vi "Dialog.vi"(8 "error in (no error)":errorcluster, 10 "Scripts Dir":path, 11 "Definitions in":T1) -> (0 "error out":errorcluster, 2 "commit?":bool, 3 "Definitions out":T1)   [LabVIEW 2019, in "Script.lvlib"]
doc: "Help dialog to configure script shortctus.\n\nCreated by: Ryan Pacini"
uses:
  Script.lvlib
  Definitions.ctl
panel:
  in  "open_qd_vi":bool
  in  "Cancel":bool
  in  "OK":bool
  in  "tab":enum32{"Help", "Script Shortcuts"}(tab)
  in  "info":string="Instructions:\n  Enter one or more script shortcuts (separated by a space) into\n  the Quick Drop textbox to execute a series of actions on the\n  selected front panel or block diagram objects.\n\nUsage: Ctrl-Space + \"<shortcut>\" + Ctrl-S"
  in  "Script Help":u16(ring) items=["Select VI...", "Builtins.vi", "TestScript.vi"]
  out "Description":string
  out "Scripts:":string
  in  "Show VI Info":bool
  in  "Shortcut":string
  in  "Action":u16(ring) items=["None", "Align Bottom Edges", "Align Horizontal Centers", "Align Left Edges", "Align Right Edges", "Align Top Edges", "Align Vertical Centers", "Arrange", "Change to CDB", "Change to CSG", "Change to CXT", "Change to DBL", "Change to EXT", "Change to I16", "Change to I32", "Change to I64", "Change to I8", "Change to SGL", "Change to U16", "Change to U32", "Change to U64", "Change to U8", "Cluster Size Fit", "Cluster Size Horizontally", "Cluster Size None", "Cluster Size Vertically", "Connect Pane", "Distribute Bottom Edges", "Distribute Horizontal Centers", "Distribute Horizontal Compress", "Distribute Horizontal Gap", "Distribute Left Edges", "Distribute Right Edges", "Distribute Top Edges", "Distribute Vertical Centers", "Distribute Vertical Compress", "Distribute Vertical Gap", "Edit Library Icon", "Error Structure", "Hide Caption", "Hide Inc/Dec Buttons", "Hide Index Display", "Hide Label", "Hide Radix", "Hide Scrollbars", "Merge Icon Layers", "My Custom Shortcut", "My Custom Shortcut with Args", "Open in File Explore", "Radix Binary or Backslash", "Radix Decimal or Normal", "Radix Hex", "Rename Caption", "Rename Label", "Reset Panel Origins", "Resizes Window", "Select Controls", "Select Controls and Indicators", "Select Indicators", "Select None", "Show Caption", "Show Inc/Dec Buttons", "Show Index Display", "Show Label", "Show Scrollbars", "Snap to Panel Grid", "VI Voodoo"]
  in  "add":bool
  in  "Script Shortcuts":i32[](listbox)
  in  "remove_shortcuts":bool
  in  "remove_all":bool
  in  "restore_defaults":bool
  in  "remove_action":bool
  in  "Actions":i32(listbox)
  in  "move_up":bool
  in  "move_down":bool
  # "Add Shortcut"
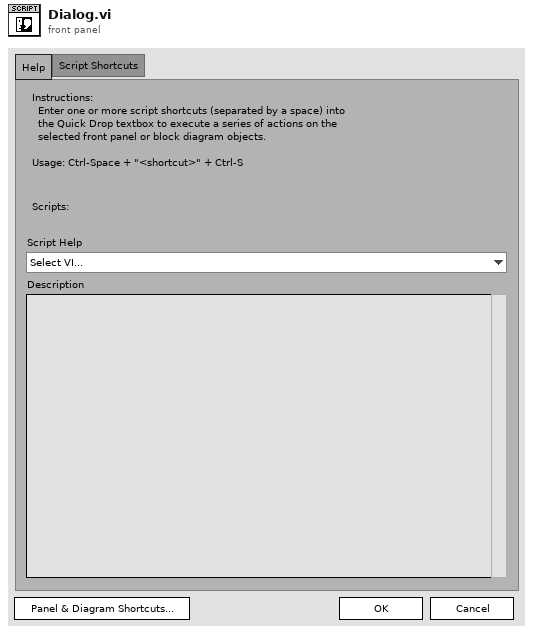
[diagram p1: front panel]
types:
  T1 = typedef "Script.lvlib/Definitions.ctl" = cluster{"plugins":cluster{"vi":path, "desc":string}[], "defaults":cluster{"uid":string, "name":string}[], "shortcuts":cluster{"shortcut":string, "uids":string[]}[], "defaults?":bool}
  T2 = cluster{"defs":T1, "ScriptsDir":path, "_sc":string, "_uid":string, "_show_uids":bool, "_action_idx":i32}
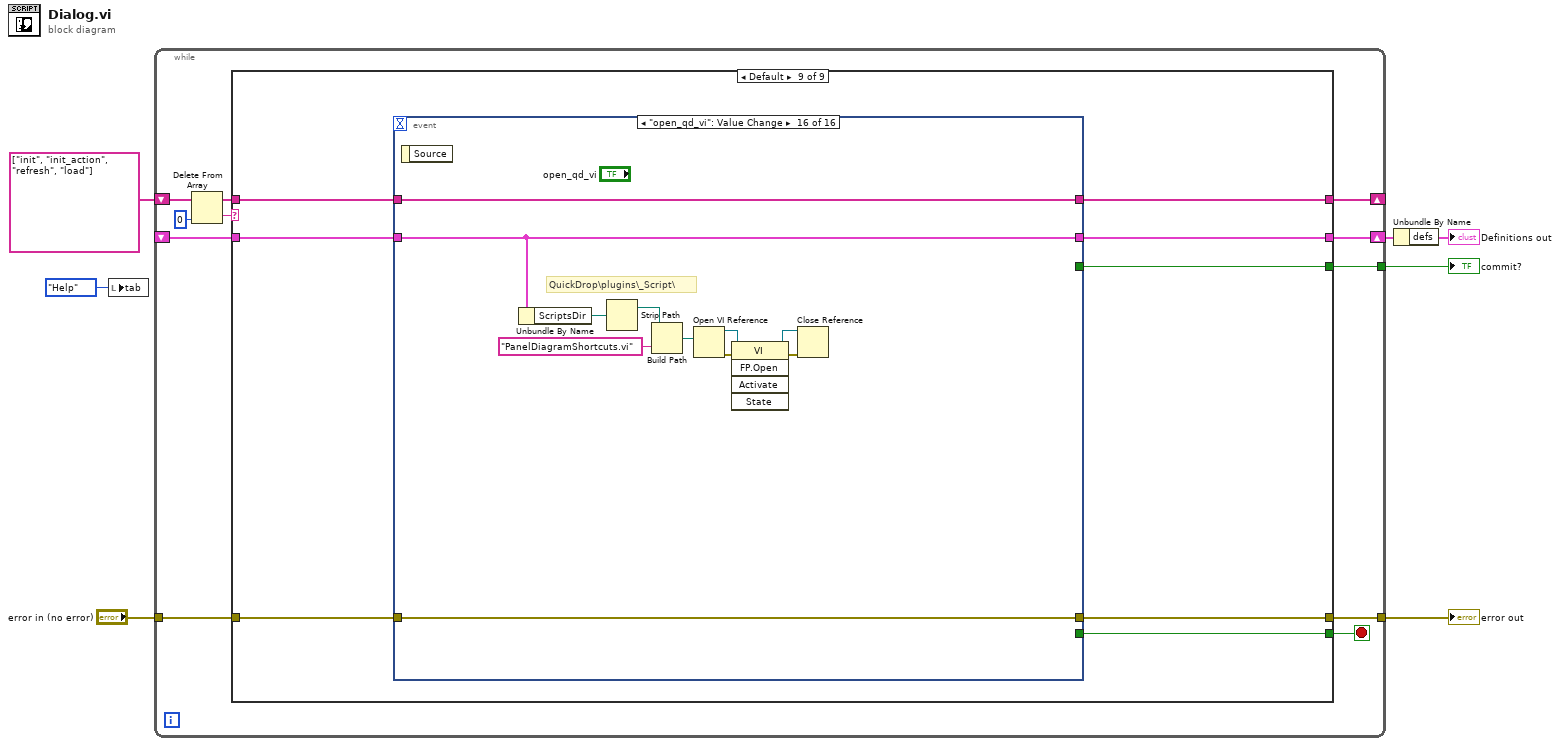
[diagram p0: block diagram]
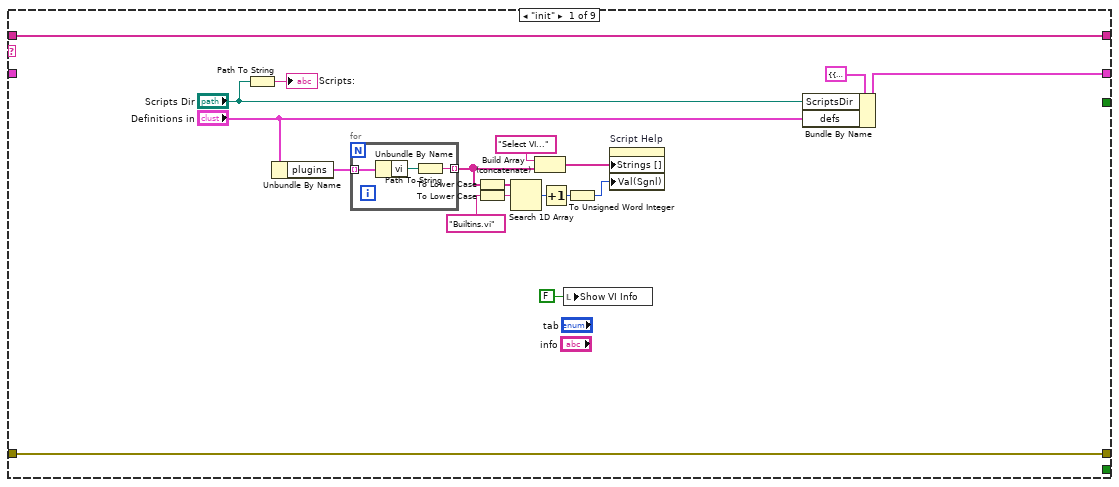
[diagram p2: hidden frame]
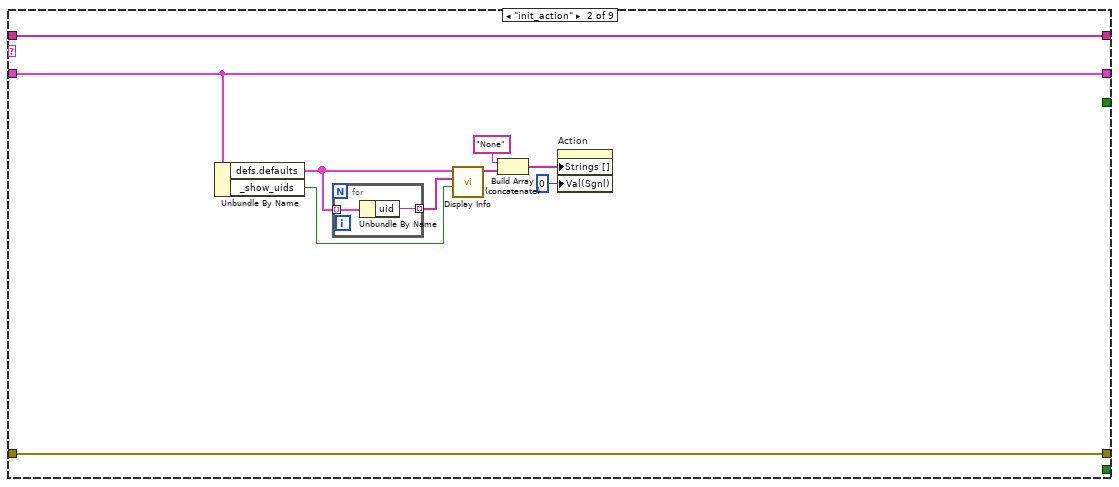
[diagram p3: hidden frame]
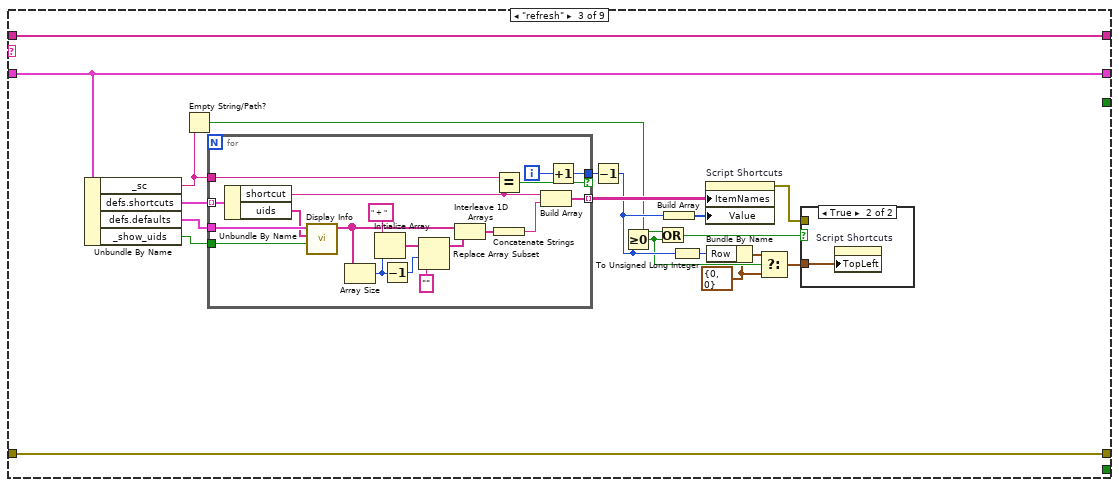
[diagram p4: hidden frame]
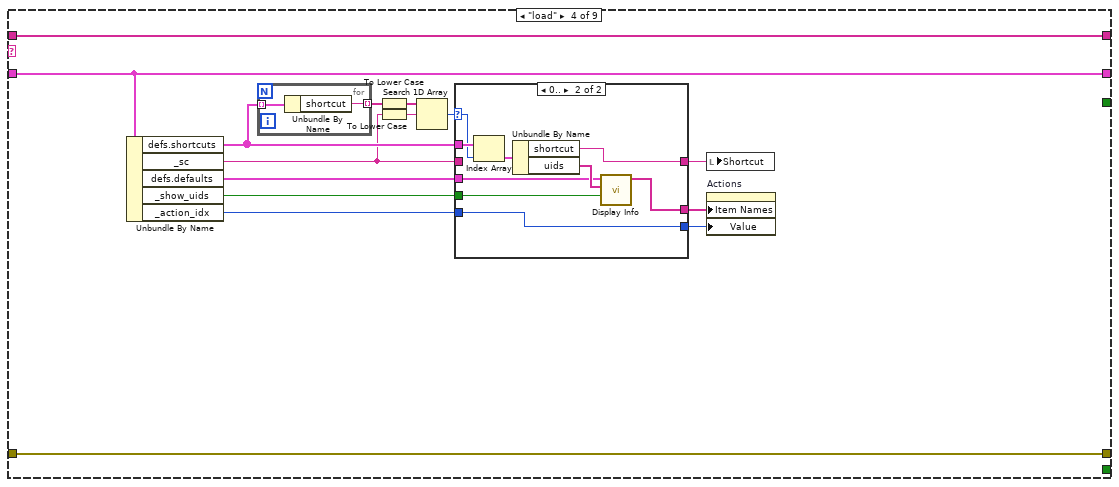
[diagram p6: hidden frame]
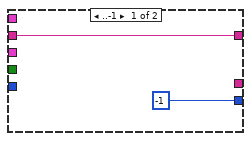
[diagram p7: hidden frame]
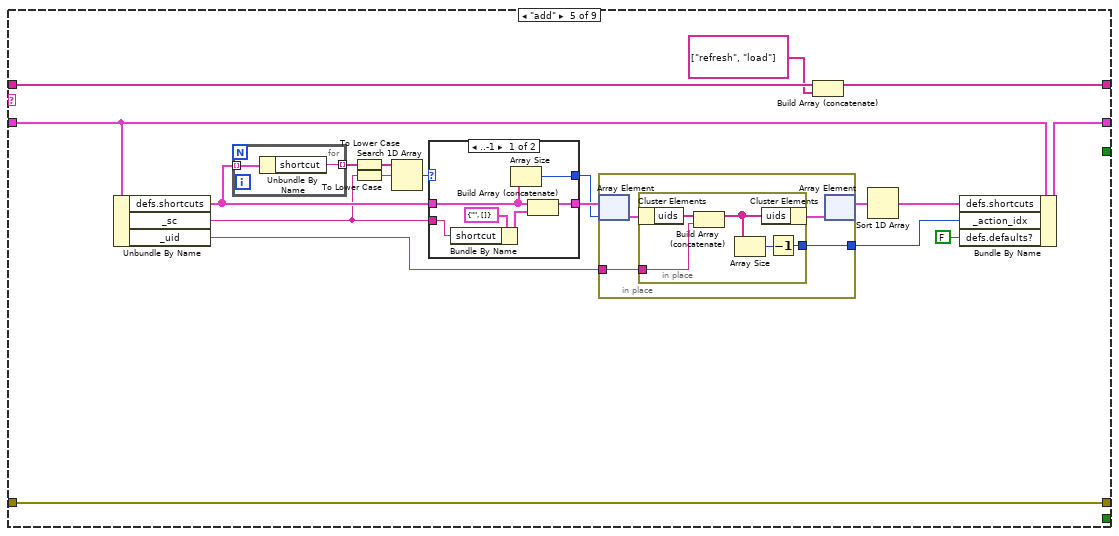
[diagram p8: hidden frame]
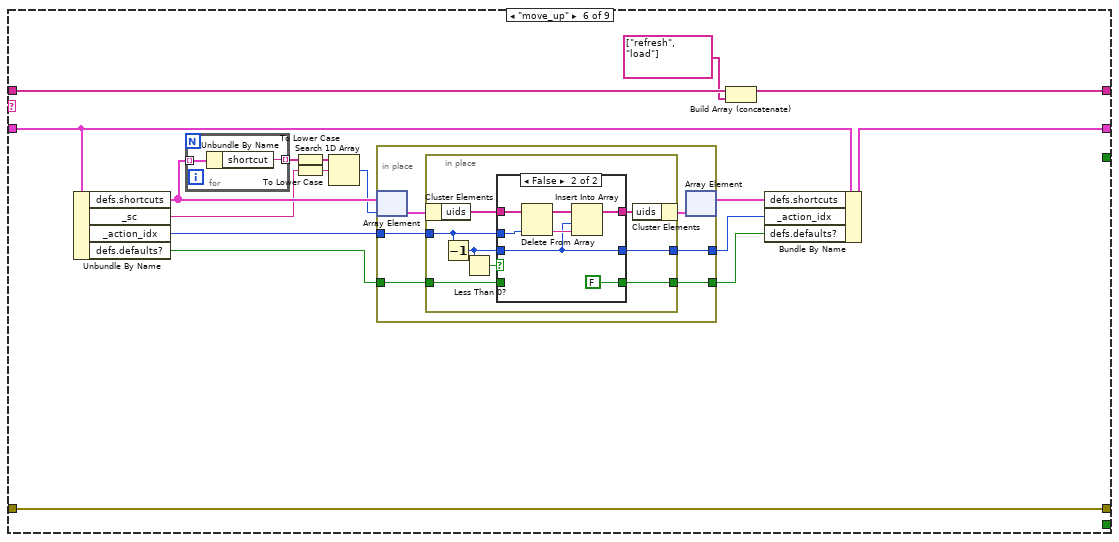
[diagram p10: hidden frame]
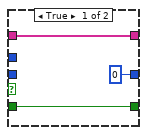
[diagram p11: hidden frame]
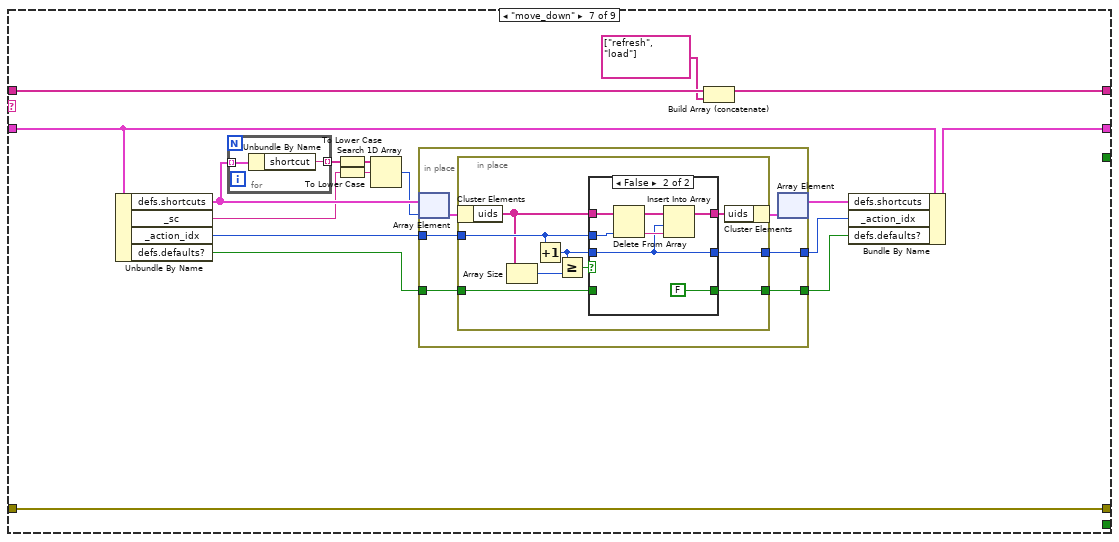
[diagram p12: hidden frame]
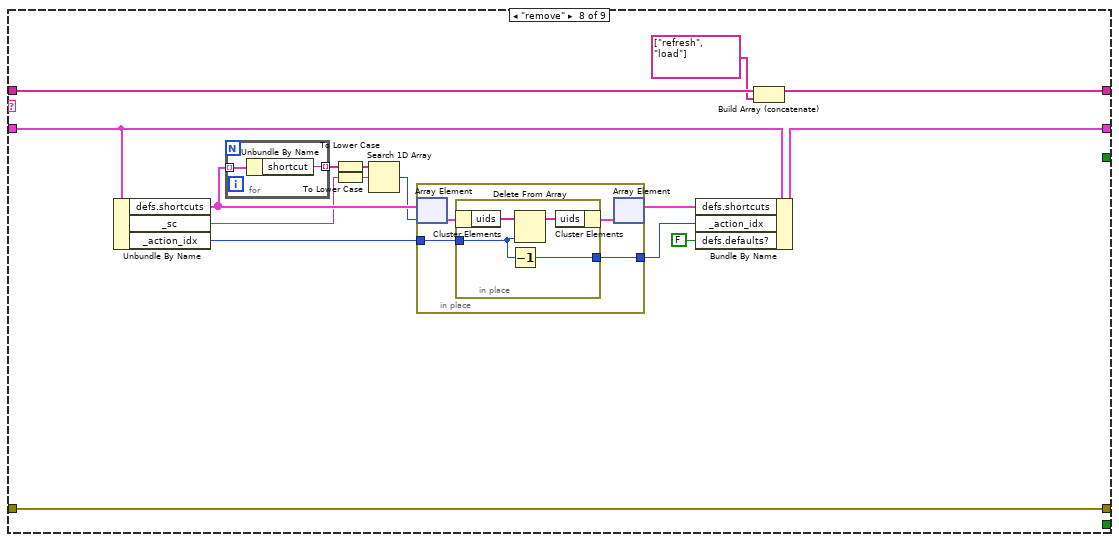
[diagram p14: hidden frame]
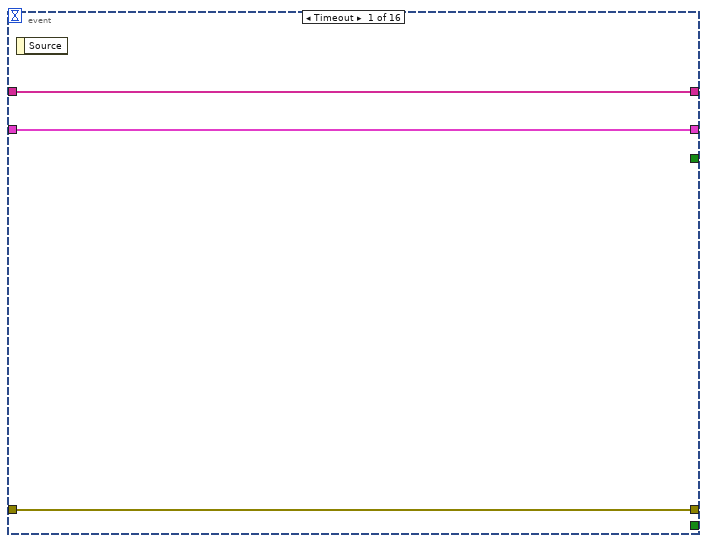
[diagram p15: hidden frame]
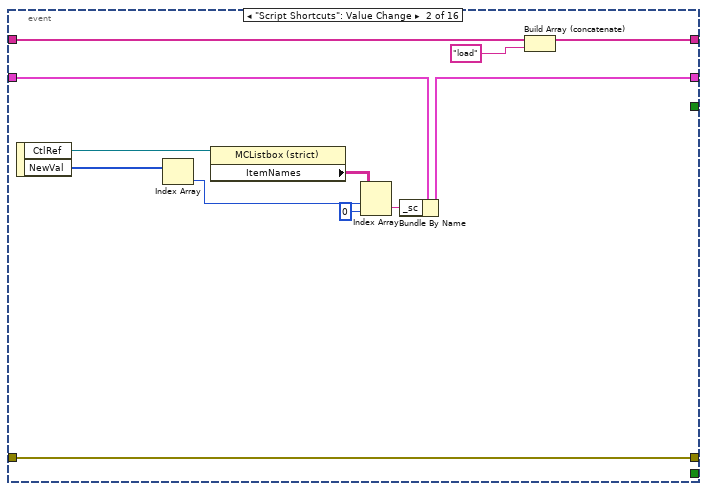
[diagram p16: hidden frame]
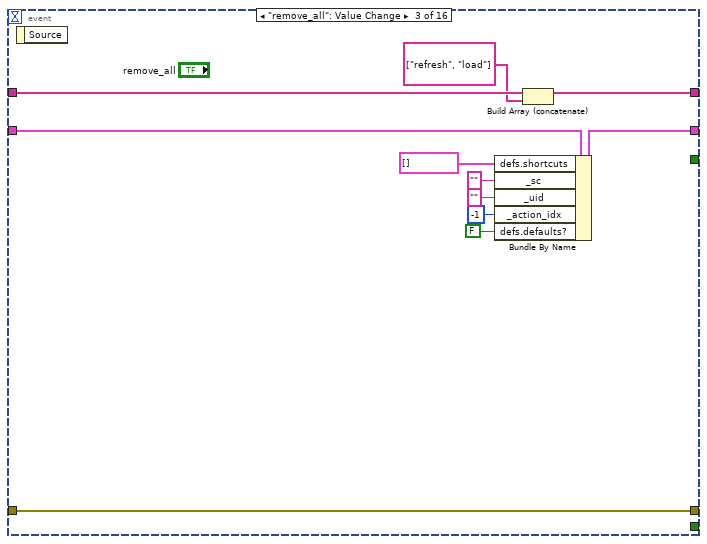
[diagram p17: hidden frame]
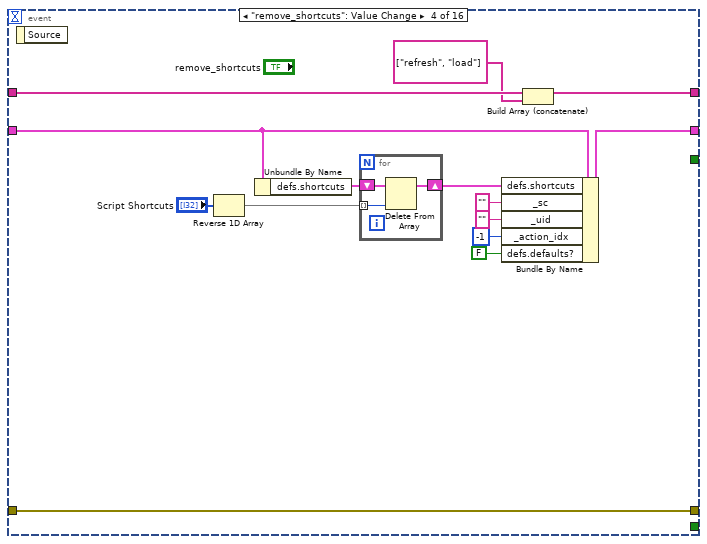
[diagram p18: hidden frame]
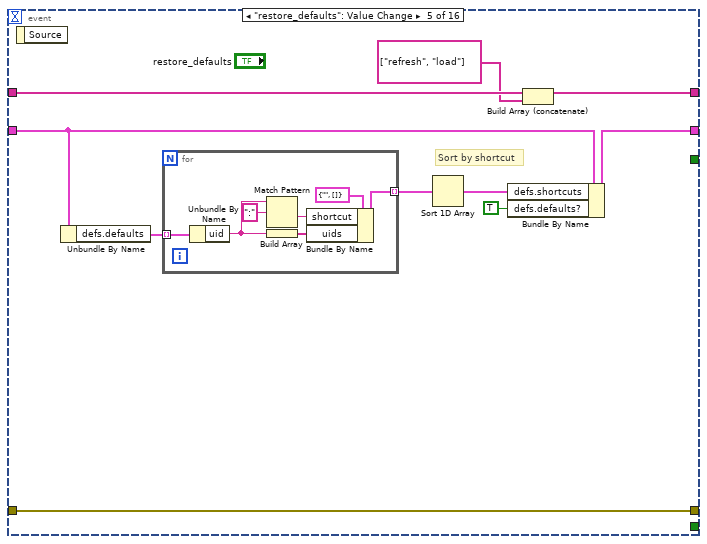
[diagram p19: hidden frame]
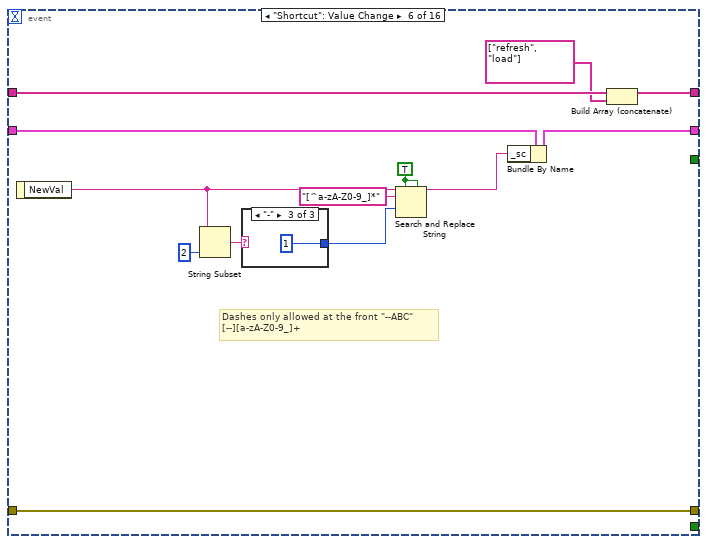
[diagram p20: hidden frame]
diagram:
  n1 = local write "tab"(enum32{"Help", "Script Shortcuts"}."Help" ("tab")) -> ()
  n2 = while {
    tunnel: [w17] -> w6
    tunnel: "error in (no error)" -> [w16]
    shift-right: [w10] -> _
    shift-left: string[] ["init", "init_action", "refresh", "load"] -> [w15]
    shift-right: [w12] -> w3
    shift-left: _ -> [w11]
    tunnel: [w8] -> w4
    stop <- w18 stop-if-true
    n3 = Delete From Array(array=w15, index=0) -> (deleted portion=w14:string, array with subset deleted=w13:string[])  [unwired: 1 in]
    n4 = case shown="Default" w14 {
      tunnel: [_ _ _ _ _ _ _ _ w277] -> w18
      tunnel: [w34 w49 w70 w105 w137 w173 w216 w259 w276] -> w17
      tunnel: w16 -> [w34 w49 w70 w105 w137 w173 w216 w259 w275]
      tunnel: w13 -> [w35 w48 w69 w104 w136 w172 w215 w258 w271]
      tunnel: [w36 w47 w68 w103 w134 w170 w202 w245 w274] -> w12
      tunnel: w11 -> [_ w47 w68 w103 w135 w171 w203 w246 w273]
      tunnel: [w35 w48 w69 w104 w123 w169 w214 w257 w272] -> w10
      tunnel: [_ _ _ _ _ _ _ _ w270] -> w8
      frame "init" {
        n5 = Path To String(path="Scripts Dir") -> (string=→"Scripts:":string)
        n6 = Unbundle By Name("Definitions in") -> ("plugins"=w30:cluster{"vi":path, "desc":string}[])
        n7 = for {
          tunnel: w30 -> [w39] mode=indexing
          tunnel: [w37] -> w27 mode=indexing
          n8 = Unbundle By Name(w39) -> ("vi"=w38:path)
          n9 = Path To String(path=w38) -> (string=w37:string)
        }
        n10 = To Lower Case(string=w27) -> (all lower case string=w24:string[])
        n11 = To Lower Case(string="Builtins.vi" ("element")) -> (all lower case string=w25:string)
        n12 = Search 1D Array(1D array=w24, element=w25) -> (index of element=w21:i32)  [unwired: 1 in]
        n13 = Build Array (concatenate)("Select VI...", w27) -> (w23:string[])
        n14 = Increment(x=w21) -> (x+1=w20:i32)
        n15 = local write "Show VI Info"(FALSE ("Show VI Info")) -> ()
        n16 = To Unsigned Word Integer(number=w20) -> (unsigned 16bit integer=w19:u16)
        n17 = property on="Script Help" class="Ring (strict)"("Strings []"=w23, "Val(Sgnl)"=w19) -> ()  [unwired: 2 in, 2 out]
        n18 = Bundle By Name(cluster=T2 {"defs"={"plugins"=[], "defaults"=[], "shortcuts"=[], "defaults?"=FALSE}, "ScriptsDir"=path "", "_sc"="", "_uid"="", "_show_uids"=FALSE, "_action_idx"=0} ("internal"), "ScriptsDir"="Scripts Dir", "defs"="Definitions in") -> (w36:T2)
      }
      frame "init_action" {
        n19 = Unbundle By Name(w47) -> ("defs.defaults"=w42:cluster{"uid":string, "name":string}[], "_show_uids"=w41:bool)
        n20 = for {
          tunnel: w42 -> [w51] mode=indexing
          tunnel: [w50] -> w43 mode=indexing
          n21 = Unbundle By Name(w51) -> ("uid"=w50:string)
        }
        n22 = call "Display Info.vi"("Show uid? (F)"=w41, "uids"=w43, "defaults"=w42) -> ("display"=w40:string[])  [unwired: 8 in]
        n23 = Build Array (concatenate)("None" ("String"), w40) -> (w46:string[])
        n24 = property on="Action" class="Ring (strict)"("Strings []"=w46, "Val(Sgnl)"=u16 0 ("Value (Signaling)")) -> ()  [unwired: 2 in, 2 out]
      }
      frame "refresh" {
        w57 = cluster{"Row":u32, "Column":u32} {"Row"=0, "Column"=0} ("Top Left Visible Cell")
        n25 = Unbundle By Name(w68) -> ("_sc"=w61:string, "defs.shortcuts"=w65:cluster{"shortcut":string, "uids":string[]}[], "defs.defaults"=w53:cluster{"uid":string, "name":string}[], "_show_uids"=w64:bool)
        n26 = Empty String/Path?(string/path=w61) -> (empty?=w60:bool)
        n27 = for {
          tunnel: w65 -> [w87] mode=indexing
          tunnel: [w90] -> w67 mode=indexing
          tunnel: [w76] -> w63 if=w88
          tunnel: w61 -> [w89]
          tunnel: w64 -> [w73]
          tunnel: w53 -> [w75]
          i -> [w77]
          n28 = Unbundle By Name(w87) -> ("shortcut"=w78:string, "uids"=w74:string[])
          n29 = call "Display Info.vi"("Show uid? (F)"=w73, "uids"=w74, "defaults"=w75) -> ("display"=w72:string[])  [unwired: 8 in]
          n30 = Array Size(array=w72) -> (size(s)=w84:i32)
          n31 = Initialize Array(" + " ("delimiter (Tab)"), w84) -> (w85:string[])
          n32 = Decrement(x=w84) -> (x-1=w83:i32)
          n33 = Replace Array Subset(array=w85, new element="" ("new element/subarray"), index=w83) -> (w82:string[])
          n34 = Interleave 1D Arrays(w72, w82) -> (w80:string[])
          n35 = Equal?(x=w89, y=w78) -> (x = y?=w88:bool)
          n36 = Concatenate Strings(w80) -> (w79:string)
          n37 = Build Array(w78, w79) -> (w90:string[])
          n38 = Increment(x=w77) -> (x+1=w76:i32)
        }
        n39 = Decrement(x=w63) -> (x-1=w62:i32)
        n40 = Greater Or Equal To 0?(x=w62) -> (x >= 0?=w59:bool)
        n41 = Or(x=w60, y=w59) -> (x .or. y?=w56:bool)
        n42 = Build Array(w62) -> (w66:i32[])
        n43 = To Unsigned Long Integer(number=w62) -> (unsigned 32bit integer=w52:u32)
        n44 = property on="Script Shortcuts" class="MCListbox (strict)"("ItemNames"=w67, "Value"=w66) -> (error out=w54:errorcluster)  [unwired: 2 in, 1 out]
        n45 = Bundle By Name(cluster=w57, "Row"=w52) -> (w58:cluster{"Row":u32, "Column":u32})
        n46 = Select(t=w58, s=w59, f=w57) -> (s? t:f=w55:cluster{"Row":u32, "Column":u32})
        n47 = case shown="True" w56 {
          tunnel: w55 -> [_ w71]
          tunnel: w54 -> [_ _]
          frame False {
          }
          frame True {
            n48 = property on="Script Shortcuts" class="MCListbox (strict)"("TopLeft"=w71) -> ()  [unwired: 2 in, 2 out]
          }
        }
      }
      frame "load" {
        n49 = Unbundle By Name(w103) -> ("defs.shortcuts"=w96:cluster{"shortcut":string, "uids":string[]}[], "_sc"=w94:string, "defs.defaults"=w93:cluster{"uid":string, "name":string}[], "_show_uids"=w92:bool, "_action_idx"=w100:i32)
        n50 = for {
          tunnel: w96 -> [w107] mode=indexing
          tunnel: [w106] -> w99 mode=indexing
          n51 = Unbundle By Name(w107) -> ("shortcut"=w106:string)
        }
        n52 = To Lower Case(string=w99) -> (all lower case string=w98:string[])
        n53 = To Lower Case(string=w94) -> (all lower case string=w97:string)
        n54 = Search 1D Array(1D array=w98, element=w97) -> (index of element=w95:i32)  [unwired: 1 in]
        n55 = case shown="0.." w95 {
          selector: w95 -> [_ w116]
          tunnel: [_ w111] -> w102
          tunnel: w96 -> [_ w117]
          tunnel: [w109 w115] -> w101
          tunnel: w100 -> [_ w110]
          tunnel: w94 -> [w109 _]
          tunnel: w93 -> [_ w113]
          tunnel: w92 -> [_ w112]
          tunnel: [-1 ("idx") w110] -> w91
          frame ..-1 {
          }
          frame 0.. {
            n56 = Index Array(array=w117, index=w116) -> (element=w118:cluster{"shortcut":string, "uids":string[]})
            n57 = Unbundle By Name(w118) -> ("shortcut"=w115:string, "uids"=w114:string[])
            n58 = call "Display Info.vi"("Show uid? (F)"=w112, "uids"=w114, "defaults"=w113) -> ("display"=w111:string[])  [unwired: 8 in]
          }
        }
        n59 = local write "Shortcut"(w101) -> ()
        n60 = property on="Actions" class="LstBox (strict)"("Item Names"=w102, "Value"=w91) -> ()  [unwired: 2 in, 2 out]
      }
      frame "add" {
        n61 = Unbundle By Name(w135) -> ("defs.shortcuts"=w129:cluster{"shortcut":string, "uids":string[]}[], "_sc"=w126:string, "_uid"=w125:string)
        n62 = for {
          tunnel: w129 -> [w156] mode=indexing
          tunnel: [w155] -> w133 mode=indexing
          n63 = Unbundle By Name(w156) -> ("shortcut"=w155:string)
        }
        n64 = To Lower Case(string=w133) -> (all lower case string=w132:string[])
        n65 = To Lower Case(string=w126) -> (all lower case string=w131:string)
        n66 = Search 1D Array(1D array=w132, element=w131) -> (index of element=w130:i32)  [unwired: 1 in]
        n67 = case shown="..-1" w130 {
          selector: w130 -> [_ w153]
          tunnel: [w152 w154] -> w128
          tunnel: w129 -> [w148 w154]
          tunnel: [w147 w153] -> w127
          tunnel: w126 -> [w149 _]
          frame ..-1 {
            n68 = Bundle By Name(cluster=cluster{"shortcut":string, "uids":string[]} {"shortcut"="", "uids"=[]} ("defs.shortcuts"), "shortcut"=w149) -> (w150:cluster{"shortcut":string, "uids":string[]})
            n69 = Array Size(array=w148) -> (size(s)=w147:i32)
            n70 = Build Array (concatenate)(w148, w150) -> (w152:cluster{"shortcut":string, "uids":string[]}[])
          }
          frame 0.. {
          }
        }
        n71 = in-place {
          in-place-border: w125 -> [w140]
          in-place-border: [w138] -> w121
          n72 = in-place-array #1(w128, w127) -> (w141:cluster{"shortcut":string, "uids":string[]})
          n73 = in-place {
            in-place-border: w140 -> [w145]
            in-place-border: [w142] -> w138
            n74 = in-place-cluster #2(w141) -> ("uids"=w146:string[])
            n75 = Build Array (concatenate)(w146, w145) -> (w144:string[])
            n76 = Array Size(array=w144) -> (size(s)=w143:i32)
            n77 = in-place-cluster #2("uids"=w144) -> (w139:cluster{"shortcut":string, "uids":string[]})
            n78 = Decrement(x=w143) -> (x-1=w142:i32)
          }
          n79 = in-place-array #1(w139) -> (w124:cluster{"shortcut":string, "uids":string[]}[])  [unwired: 1 out]
        }
        n80 = Build Array (concatenate)(w136, string[] ["refresh", "load"]) -> (w123:string[])
        n81 = Sort 1D Array(array=w124) -> (sorted array=w119:cluster{"shortcut":string, "uids":string[]}[])
        n82 = Bundle By Name(cluster=w135, "defs.shortcuts"=w119, "_action_idx"=w121, "defs.defaults?"=FALSE) -> (w134:T2)
      }
      frame "move_up" {
        n83 = Unbundle By Name(w171) -> ("defs.shortcuts"=w167:cluster{"shortcut":string, "uids":string[]}[], "_sc"=w165:string, "_action_idx"=w162:i32, "defs.defaults?"=w158:bool)
        n84 = for {
          tunnel: w167 -> [w175] mode=indexing
          tunnel: [w174] -> w168 mode=indexing
          n85 = Unbundle By Name(w175) -> ("shortcut"=w174:string)
        }
        n86 = To Lower Case(string=w168) -> (all lower case string=w160:string[])
        n87 = To Lower Case(string=w165) -> (all lower case string=w159:string)
        n88 = Search 1D Array(1D array=w160, element=w159) -> (index of element=w166:i32)  [unwired: 1 in]
        n89 = in-place {
          in-place-border: w162 -> [w179]
          in-place-border: [w178] -> w161
          in-place-border: w158 -> [w177]
          in-place-border: [w176] -> w157
          n90 = in-place-array #3(w167, w166) -> (w181:cluster{"shortcut":string, "uids":string[]})
          n91 = in-place {
            in-place-border: w179 -> [w186]
            in-place-border: [w187] -> w178
            in-place-border: w177 -> [w183]
            in-place-border: [w182] -> w176
            n92 = in-place-cluster #4(w181) -> ("uids"=w189:string[])
            n93 = Decrement(x=w186) -> (x-1=w185:i32)
            n94 = Less Than 0?(x=w185) -> (x < 0?=w184:bool)
            n95 = case shown="False" w184 {
              tunnel: w189 -> [w192 w198]
              tunnel: [w192 w197] -> w188
              tunnel: [0 w194] -> w187
              tunnel: w186 -> [_ w196]
              tunnel: w185 -> [_ w194]
              tunnel: w183 -> [w190 _]
              tunnel: [w190 FALSE ("defaults?")] -> w182
              frame True {
              }
              frame False {
                n96 = Delete From Array(array=w198, index=w196) -> (deleted portion=w195:string, array with subset deleted=w199:string[])  [unwired: 1 in]
                n97 = Insert Into Array(array=w199, index=w194, new element=w195) -> (w197:string[])
              }
            }
            n98 = in-place-cluster #4("uids"=w188) -> (w180:cluster{"shortcut":string, "uids":string[]})
          }
          n99 = in-place-array #3(w180) -> (w163:cluster{"shortcut":string, "uids":string[]}[])  [unwired: 1 out]
        }
        n100 = Build Array (concatenate)(w172, string[] ["refresh", "load"]) -> (w169:string[])
        n101 = Bundle By Name(cluster=w171, "defs.shortcuts"=w163, "_action_idx"=w161, "defs.defaults?"=w157) -> (w170:T2)
      }
      frame "move_down" {
        n102 = Unbundle By Name(w203) -> ("defs.shortcuts"=w211:cluster{"shortcut":string, "uids":string[]}[], "_sc"=w209:string, "_action_idx"=w207:i32, "defs.defaults?"=w201:bool)
        n103 = for {
          tunnel: w211 -> [w218] mode=indexing
          tunnel: [w217] -> w212 mode=indexing
          n104 = Unbundle By Name(w218) -> ("shortcut"=w217:string)
        }
        n105 = To Lower Case(string=w212) -> (all lower case string=w205:string[])
        n106 = To Lower Case(string=w209) -> (all lower case string=w204:string)
        n107 = Search 1D Array(1D array=w205, element=w204) -> (index of element=w210:i32)  [unwired: 1 in]
        n108 = in-place {
          in-place-border: w207 -> [w222]
          in-place-border: [w221] -> w206
          in-place-border: [w220] -> w200
          in-place-border: w201 -> [w219]
          n109 = in-place-array #5(w211, w210) -> (w224:cluster{"shortcut":string, "uids":string[]})
          n110 = in-place {
            in-place-border: w222 -> [w231]
            in-place-border: [w232] -> w221
            in-place-border: [w226] -> w220
            in-place-border: w219 -> [w225]
            n111 = in-place-cluster #6(w224) -> ("uids"=w228:string[])
            n112 = Array Size(array=w228) -> (size(s)=w227:i32)
            n113 = Increment(x=w231) -> (x+1=w230:i32)
            n114 = Greater Or Equal?(x=w230, y=w227) -> (x >= y?=w229:bool)
            n115 = case shown="False" w229 {
              tunnel: w228 -> [w236 w242]
              tunnel: [w236 w241] -> w233
              tunnel: [w235 w238] -> w232
              tunnel: w231 -> [w235 w240]
              tunnel: w230 -> [_ w238]
              tunnel: [w234 FALSE ("defaults?")] -> w226
              tunnel: w225 -> [w234 _]
              frame True {
              }
              frame False {
                n116 = Delete From Array(array=w242, index=w240) -> (deleted portion=w239:string, array with subset deleted=w243:string[])  [unwired: 1 in]
                n117 = Insert Into Array(array=w243, index=w238, new element=w239) -> (w241:string[])
              }
            }
            n118 = in-place-cluster #6("uids"=w233) -> (w223:cluster{"shortcut":string, "uids":string[]})
          }
          n119 = in-place-array #5(w223) -> (w208:cluster{"shortcut":string, "uids":string[]}[])  [unwired: 1 out]
        }
        n120 = Build Array (concatenate)(w215, string[] ["refresh", "load"]) -> (w214:string[])
        n121 = Bundle By Name(cluster=w203, "defs.shortcuts"=w208, "_action_idx"=w206, "defs.defaults?"=w200) -> (w202:T2)
      }
      frame "remove" {
        n122 = Unbundle By Name(w246) -> ("defs.shortcuts"=w254:cluster{"shortcut":string, "uids":string[]}[], "_sc"=w252:string, "_action_idx"=w250:i32)
        n123 = for {
          tunnel: w254 -> [w261] mode=indexing
          tunnel: [w260] -> w255 mode=indexing
          n124 = Unbundle By Name(w261) -> ("shortcut"=w260:string)
        }
        n125 = To Lower Case(string=w255) -> (all lower case string=w248:string[])
        n126 = To Lower Case(string=w252) -> (all lower case string=w247:string)
        n127 = Search 1D Array(1D array=w248, element=w247) -> (index of element=w253:i32)  [unwired: 1 in]
        n128 = in-place {
          in-place-border: w250 -> [w263]
          in-place-border: [w262] -> w249
          n129 = in-place-array #7(w254, w253) -> (w265:cluster{"shortcut":string, "uids":string[]})
          n130 = in-place {
            in-place-border: w263 -> [w267]
            in-place-border: [w266] -> w262
            n131 = in-place-cluster #8(w265) -> ("uids"=w269:string[])
            n132 = Decrement(x=w267) -> (x-1=w266:i32)
            n133 = Delete From Array(array=w269, index=w267) -> (array with subset deleted=w268:string[])  [unwired: 1 in, 1 out]
            n134 = in-place-cluster #8("uids"=w268) -> (w264:cluster{"shortcut":string, "uids":string[]})
          }
          n135 = in-place-array #7(w264) -> (w251:cluster{"shortcut":string, "uids":string[]}[])  [unwired: 1 out]
        }
        n136 = Bundle By Name(cluster=w246, "defs.shortcuts"=w251, "_action_idx"=w249, "defs.defaults?"=FALSE) -> (w245:T2)
        n137 = Build Array (concatenate)(w258, string[] ["refresh", "load"]) -> (w257:string[])
      }
      frame Default {
        n138 = event shown="[15] \"open_qd_vi\": Value Change" {
          selector: _ -> [_ _ _ _ _ _ _ _ _ _ _ _ _ _ _ _]
          dyn-events: _ -> [_ _ _ _ _ _ _ _ _ _ _ _ _ _ _ _]
          timeout: _ -> [_ _ _ _ _ _ _ _ _ _ _ _ _ _ _ _]
          tunnel: [_ _ _ _ _ _ _ _ _ _ _ TRUE TRUE _ _ _] -> w277
          tunnel: [w280 w292 w303 w317 w330 w350 w363 w383 w388 w393 w398 w401 w407 w417 w426 w437] -> w276
          tunnel: w275 -> [w280 w292 w303 w317 w330 w350 w363 w383 w388 w393 w398 w401 w407 w417 w426 w437]
          tunnel: [w278 w289 w299 w312 w326 w348 w360 w381 w387 w392 w397 w399 w406 w415 w423 w435] -> w274
          tunnel: w273 -> [w278 w291 w294 w311 w325 w344 w361 w380 w387 w392 w397 w399 w406 w415 w425 w435]
          tunnel: [w279 w287 w301 w315 w328 w347 w359 w382 w385 w390 w395 w400 w405 w416 w421 w436] -> w272
          tunnel: w271 -> [w279 w290 w302 w316 w329 w349 w362 w382 w386 w391 w396 w400 w405 w416 w424 w436]
          tunnel: [_ _ _ _ _ _ _ _ _ _ _ _ TRUE _ _ _] -> w270
          event Timeout {
            n139 = event-data() -> ()  [unwired: 1 in, 1 out]
          }
          event "Script Shortcuts": Value Change {
            n140 = event-data() -> ("CtlRef"=w285:refnum<vi>, "NewVal"=w288:i32[])  [unwired: 1 in]
            n141 = Index Array(array=w288) -> (element=w283:i32)  [unwired: 1 in]
            n142 = property class="MCListbox (strict)"(reference=w285) -> ("ItemNames"=w284:string[][])  [unwired: 1 in, 2 out]
            n143 = Index Array(array=w284, index (row)=w283, index (col)=0 ("disabled index (col)")) -> (element=w281:string)
            n144 = Bundle By Name(cluster=w291, "_sc"=w281) -> (w289:T2)
            n145 = Build Array (concatenate)(w290, "load") -> (w287:string[])
          }
          event "remove_all": Value Change {
            n146 = event-data() -> ()  [unwired: 1 in, 1 out]
            n147 = Bundle By Name(cluster=w294, "defs.shortcuts"=cluster{"shortcut":string, "uids":string[]}[] [], "_sc"="", "_uid"="", "_action_idx"=-1, "defs.defaults?"=FALSE) -> (w299:T2)
            n148 = Build Array (concatenate)(w302, string[] ["refresh", "load"]) -> (w301:string[])
          }
          event "remove_shortcuts": Value Change {
            n149 = event-data() -> ()  [unwired: 1 in, 1 out]
            n150 = Reverse 1D Array(array="Script Shortcuts") -> (reversed array=w310:i32[])
            n151 = Unbundle By Name(w311) -> ("defs.shortcuts"=w309:cluster{"shortcut":string, "uids":string[]}[])
            n152 = for {
              shift-right: [w318] -> w308
              shift-left: w309 -> [w320]
              tunnel: w310 -> [w319] mode=indexing
              n153 = Delete From Array(array=w320, index=w319) -> (array with subset deleted=w318:cluster{"shortcut":string, "uids":string[]}[])  [unwired: 1 in, 1 out]
            }
            n154 = Bundle By Name(cluster=w311, "defs.shortcuts"=w308, "_sc"="", "_uid"="", "_action_idx"=-1, "defs.defaults?"=FALSE) -> (w312:T2)
            n155 = Build Array (concatenate)(w316, string[] ["refresh", "load"]) -> (w315:string[])
          }
          event "restore_defaults": Value Change {
            # "Sort by shortcut"
            n156 = event-data() -> ()  [unwired: 1 in, 1 out]
            n157 = Unbundle By Name(w325) -> ("defs.defaults"=w324:cluster{"uid":string, "name":string}[])
            n158 = for {
              tunnel: [w331] -> w322 mode=indexing
              tunnel: w324 -> [w336] mode=indexing
              n159 = Unbundle By Name(w336) -> ("uid"=w334:string)
              n160 = Match Pattern(string=w334, regular expression=":") -> (after substring=w332:string)  [unwired: 1 in, 3 out]
              n161 = Build Array(w334) -> (w335:string[])
              n162 = Bundle By Name(cluster=cluster{"shortcut":string, "uids":string[]} {"shortcut"="", "uids"=[]} ("defs.shortcuts"), "shortcut"=w332, "uids"=w335) -> (w331:cluster{"shortcut":string, "uids":string[]})
            }
            n163 = Sort 1D Array(array=w322) -> (sorted array=w321:cluster{"shortcut":string, "uids":string[]}[])
            n164 = Bundle By Name(cluster=w325, "defs.shortcuts"=w321, "defs.defaults?"=TRUE) -> (w326:T2)
            n165 = Build Array (concatenate)(w329, string[] ["refresh", "load"]) -> (w328:string[])
          }
          event "Shortcut": Value Change {
            w340 = TRUE ("replace all? (F)")
            # "Dashes only allowed at the front \"--ABC\"\n[--][a-zA-Z0-9_]+"
            n166 = event-data() -> ("NewVal"=w343:string)  [unwired: 1 in]
            n167 = String Subset(string=w343, length (rest)=2 ("length (rest)")) -> (substring=w339:string)  [unwired: 1 in]
            n168 = case shown="\"-\"" w339 {
              tunnel: [0 ("length (rest)") 2 ("length (rest)") 1 ("length (rest)")] -> w338
              frame Default {
              }
              frame "--" {
              }
              frame "-" {
              }
            }
            n169 = Search and Replace String(replace all?=w340, multiline?=w340, input string=w343, search string="[^a-zA-Z0-9_]*", offset=w338) -> (result string=w345:string)  [unwired: 3 in, 3 out]
            n170 = Bundle By Name(cluster=w344, "_sc"=w345) -> (w348:T2)
            n171 = Build Array (concatenate)(w349, string[] ["refresh", "load"]) -> (w347:string[])
          }
          event "add": Value Change {
            n172 = event-data() -> ()  [unwired: 1 in, 1 out]
            n173 = Empty String/Path?(string/path="Shortcut") -> (empty?=w357:bool)
            n174 = Equal To 0?(x="Action") -> (x = 0?=w354:bool)
            n175 = Or(x=w357, y=w354) -> (x .or. y?=w356:bool)
            n176 = case shown="False" w356 {
              tunnel: w362 -> [w375 w378]
              tunnel: w361 -> [w370 w377]
              tunnel: [w372 w377] -> w360
              tunnel: [w374 w378] -> w359
              tunnel: "Shortcut" -> [w371 _]
              tunnel: "Action" -> [w368 _]
              frame False {
                n177 = Unbundle By Name(w370) -> ("defs.defaults"=w369:cluster{"uid":string, "name":string}[])
                n178 = To Long Integer(number=w368) -> (32bit integer=w366:i32)
                n179 = Build Array (concatenate)(w375, "add") -> (w374:string[])
                n180 = Decrement(x=w366) -> (x-1=w367:i32)
                n181 = Index Array(array=w369, index=w367) -> (element=w365:cluster{"uid":string, "name":string})
                n182 = Unbundle By Name(w365) -> ("uid"=w364:string)
                n183 = Bundle By Name(cluster=w370, "_sc"=w371, "_uid"=w364) -> (w372:T2)
              }
              frame True {
                n184 = One Button Dialog(message="Shortcut is empty or has no action") -> ()  [unwired: 1 in, 1 out]
              }
            }
          }
          event "Actions": Value Change {
            n185 = event-data() -> ("NewVal"=w379:i32)  [unwired: 1 in]
            n186 = Bundle By Name(cluster=w380, "_action_idx"=w379) -> (w381:T2)
          }
          event "move_up": Value Change {
            n187 = event-data() -> ()  [unwired: 1 in, 1 out]
            n188 = Build Array (concatenate)(w386, "move_up" ("array")) -> (w385:string[])
          }
          event "move_down": Value Change {
            n189 = event-data() -> ()  [unwired: 1 in, 1 out]
            n190 = Build Array (concatenate)(w391, "move_down" ("array")) -> (w390:string[])
          }
          event "remove_action": Value Change {
            n191 = event-data() -> ()  [unwired: 1 in, 1 out]
            n192 = Build Array (concatenate)(w396, "remove" ("array")) -> (w395:string[])
          }
          event Panel Close; "Cancel": Value Change {
            n193 = event-data() -> ()  [unwired: 1 in, 1 out]
          }
          event "OK": Value Change {
            n194 = event-data() -> ()  [unwired: 1 in, 1 out]
          }
          event "Script Help": Value Change {
            n195 = event-data() -> ("NewVal"=w411:u16)  [unwired: 1 in]
            n196 = Unbundle By Name(w415) -> ("defs.plugins"=w414:cluster{"vi":path, "desc":string}[])
            n197 = To Long Integer(number=w411) -> (32bit integer=w412:i32)
            n198 = Decrement(x=w412) -> (x-1=w410:i32)
            n199 = for {
              tunnel: w414 -> [w419] mode=indexing
              tunnel: [w418] -> w408 mode=indexing
              n200 = Unbundle By Name(w419) -> ("desc"=w418:string)
            }
            n201 = property on="Description" class="Str"("Text.Scroll Position"=u32 0) -> ()  [unwired: 2 in, 2 out]
            n202 = Index Array(array=w408, index=w410) -> (element=→"Description":string)
          }
          event "Show VI Info": Value Change {
            n203 = event-data() -> ("NewVal"=w422:bool)  [unwired: 1 in]
            n204 = Bundle By Name(cluster=w425, "_show_uids"=w422) -> (w423:T2)
            n205 = Build Array (concatenate)(w424, string[] ["init_action", "refresh", "load"]) -> (w421:string[])
          }
          event "open_qd_vi": Value Change {
            # "QuickDrop\\plugins\\_Script\\"
            n206 = event-data() -> ()  [unwired: 1 in, 1 out]
            n207 = Unbundle By Name(w435) -> ("ScriptsDir"=w434:path)
            n208 = Strip Path(path=w434) -> (stripped path=w427:path)  [unwired: 1 out]
            n209 = Build Path(base path=w427, name or relative path="PanelDiagramShortcuts.vi") -> (appended path=w432:path)
            n210 = Open VI Reference(vi path=w432) -> (vi reference=w430:refnum<vi>, error out=w431:errorcluster)  [unwired: 5 in]
            n211 = invoke class="VI" method="FP.Open"(reference=w430, error in=w431) -> (reference out=w428:refnum<vi>, error out=w429:errorcluster)  [unwired: 3 in, 3 out]
            n212 = Close Reference(reference=w428, error in (no error)=w429) -> ()  [unwired: 1 out]
          }
        }
      }
    }
  }
  "error out" <- w6
  "commit?" <- w4
  n213 = Unbundle By Name(w3) -> ("defs"=→"Definitions out":T1)
